vi "linear fit.vi"(9 "X max":i32, 10 "X min":i32, 11 "Graph plots in":cluster{"days":i32[], "Y out":dbl[]}[](array[cluster])) -> (3 "Graph plots out":cluster{"days":i32[], "Y out":dbl[]}[](array[cluster]))   [LabVIEW 2019]
uses:
  <vilib>/Analysis/NI_AALPro.lvlib
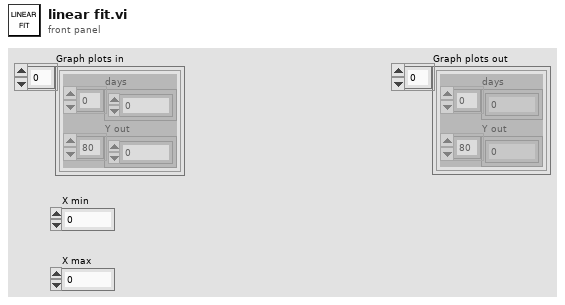
[diagram p1: front panel]
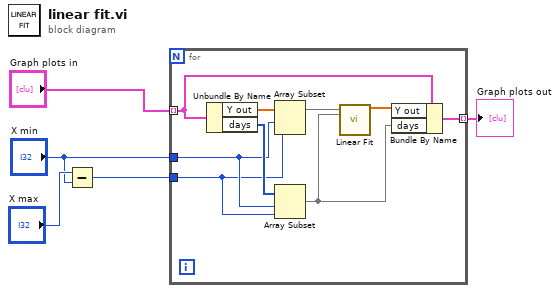
[diagram p0: block diagram]
diagram:
  n1 = Subtract(x="X max", y="X min") -> (x-y=w2:i32)
  n2 = for {
    tunnel: "Graph plots in" -> [w7] mode=indexing
    tunnel: "X min" -> [w10]
    tunnel: w2 -> [w9]
    tunnel: [w8] -> w1 mode=indexing
    n3 = Unbundle By Name(w7) -> ("Y out"=w14:dbl[], "days"=w11:i32[])
    n4 = Array Subset(array=w14, index=w10, length=w9) -> (w13:dbl[])
    n5 = Array Subset(array=w11, index=w10, length=w9) -> (w6:i32[])
    n6 = call <vilib>:"Linear Fit.vi"("Y"=w13, "X"=w6) -> ("Best Linear Fit"=w12:dbl[])  [unwired: 9 in, 4 out]
    n7 = Bundle By Name(cluster=w7, "Y out"=w12, "days"=w6) -> (w8:cluster{"days":i32[], "Y out":dbl[]})
  }
  "Graph plots out" <- w1
